vi "Main.vi"(11 "Module Admin":refnum<class "Delacor_lib_QMH_Module Admin.lvclass">) -> ()   [LabVIEW 2020, in "Sensor checking module.lvlib"]
doc: "This template is based off of the Queued Message Handler design pattern and the Queued Message Handler project template that ships with LabVIEW.\n\nThe main difference is that the queue is private to this module and communication between modules is performed via Broadcast and Request events.\n\nRequest events are wrapped in public API methods and are handled in the Event Handling Loop (EHL) of this VI. Any module can register for Broadcast events sent by this module. The EHL generates messages based on user interface actions.\n\nThe Message Handling Loop (MHL) processes messages generated by the EHL, or by other messages. The messages are string values, so new messages can be added easily to the Message Cases case structure in the MHL. Each message cluster can also provide an optional value for Message Data, which is a variant that can be converted to whatever message-specific data is required.\n_____\nBased on DQMH Project Template 7.0.1.1316."
uses:
  Sensor checking module.lvlib
  <vilib>/Delacor/Delacor QMH/Libraries/Module Admin_class/Delacor_lib_QMH_Module Admin.lvclass
  Module Data--cluster.ctl
  Simulated sensor signal HL Data.ctl
  <vilib>/Delacor/Delacor QMH/Libraries/Message Queue_class/Delacor_lib_QMH_Message Queue.lvclass/Delacor_lib_QMH_Message Queue.ctl
  Stop Argument--cluster.ctl
  <vilib>/Delacor/Delacor QMH/Libraries/Module Admin_class/Delacor_lib_QMH_Module Admin.lvclass/Delacor_lib_QMH_Module Admin.ctl
  Start sensor checking Argument--cluster.ctl
  Stop sensor checking Argument--cluster.ctl
  <vilib>/Utility/miscctls.llb/LVPointTypeDef.ctl
  <vilib>/Delacor/Delacor QMH/Libraries/Message Queue_class/Delacor_lib_QMH_Enqueue Message (Single).vi
  <vilib>/Delacor/Delacor QMH/Libraries/Module Admin_class/Delacor_lib_QMH_Get External Launch.vi
  <vilib>/Delacor/Delacor QMH/Libraries/Message Queue_class/Delacor_lib_QMH_Message Queue.lvclass
panel:
  out "error out":errorcluster
  out "Status":string
  in  "Simulate MHL Error":bool
  in  "Simulate EHL Error":bool
  # "Other processes communicate with this Module via its Public API (wrappers for its Request Events).\n\nThis Module communicates with other processes via its Broadcast Events.\nAny process that wants to receive these messages can register for this module's Broadcast events."
  # "This template is for the DQMH framework. See the block diagram for more information on how to use this template."
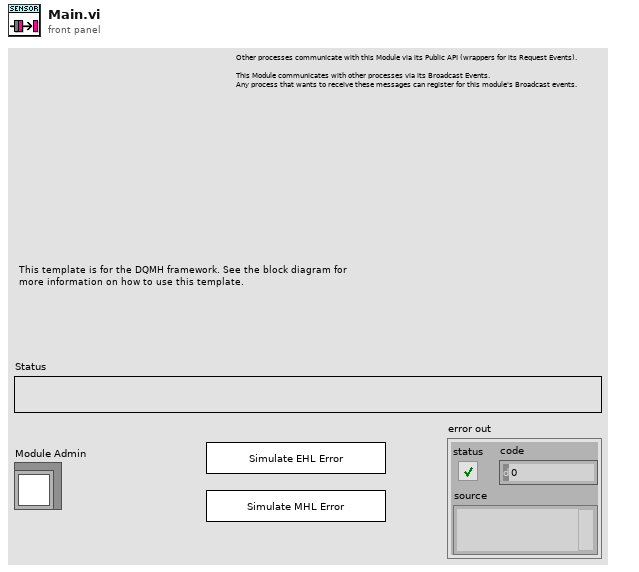
[diagram p1: front panel]
types:
  T1 = typedef "Sensor checking module.lvlib/Request Events--cluster.ctl" = cluster{"Stop Module":refnum<user-event>, "Show Panel":refnum<user-event>, "Hide Panel":refnum<user-event>, "Get Module Execution Status":refnum<user-event>, "Show Diagram":refnum<user-event>, "Start sensor checking":refnum<user-event>, "Stop sensor checking":refnum<user-event>, "Private":cluster{"Wake up HL":refnum<user-event>, "Sleep HL":refnum<user-event>}}
  T2 = typedef "Sensor checking module.lvlib/Simulated sensor signal HL Data.ctl" = cluster{"RPM increasing?":bool, "RPM":dbl}
  T3 = typedef "Sensor checking module.lvlib/Module Data--cluster.ctl" = cluster{"Status":string}
  T4 = enum32{"invalid lock state", "Not Locked", "Locked (No Password)", "Password-protected"}
  T5 = typedef "Sensor checking module.lvlib/Stop Argument--cluster.ctl" = cluster{"Origin":string, "Exit via Stop Module Req?":bool, "Wait for Module to stop?":bool}
  T6 = typedef "Sensor checking module.lvlib/Start sensor checking Argument--cluster.ctl" = cluster{"Triggered interval":dbl, "RPM increasing?":bool}
  T7 = typedef "Sensor checking module.lvlib/Stop sensor checking Argument--cluster.ctl" = cluster{"Boolean":bool}
  T8 = typedef "LVPointTypeDef.ctl" = cluster{"Horizontal":i16, "Vertical":i16}
  T9 = enum32{"Invalid", "Standard", "Closed", "Hidden", "Minimized", "Maximized"}
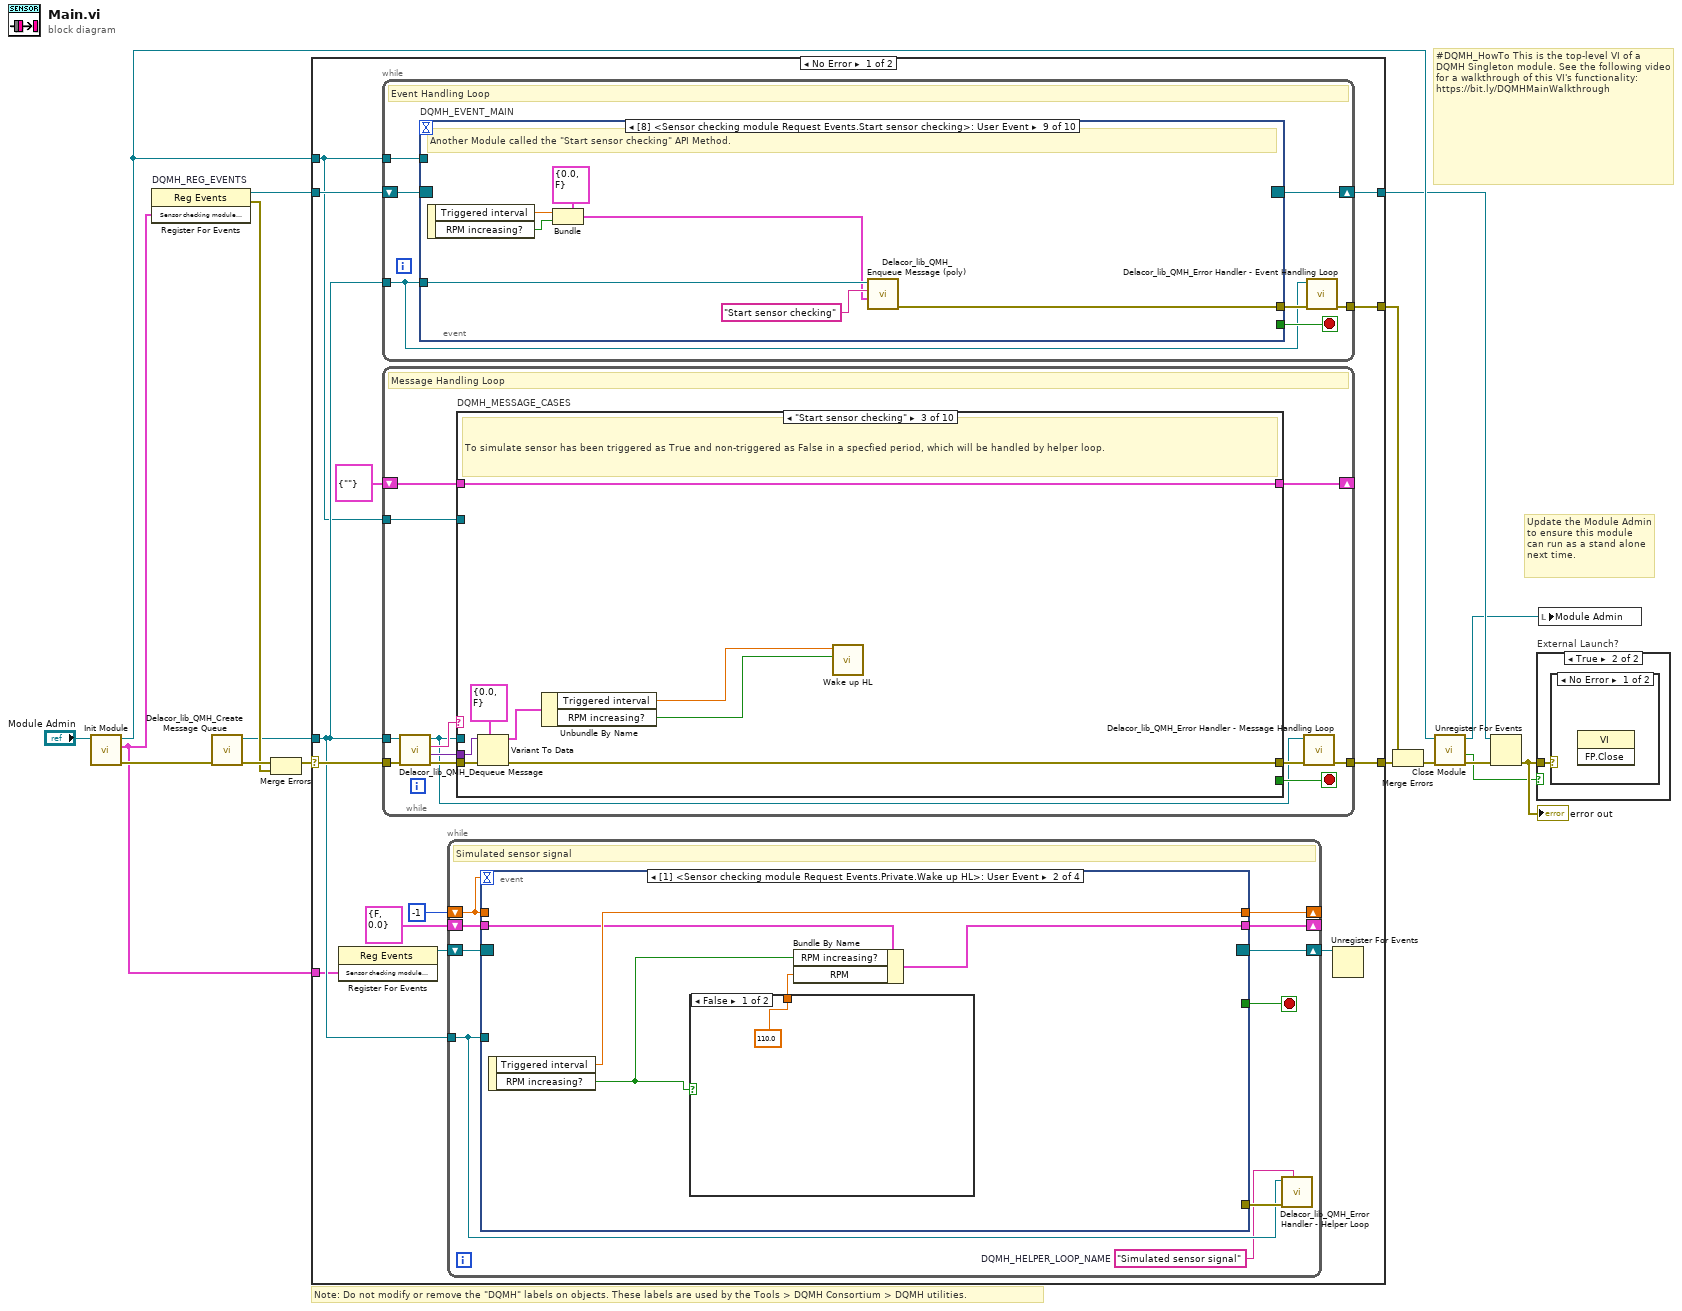
[diagram p0: block diagram]
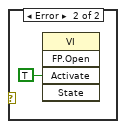
[diagram p3: hidden frame]
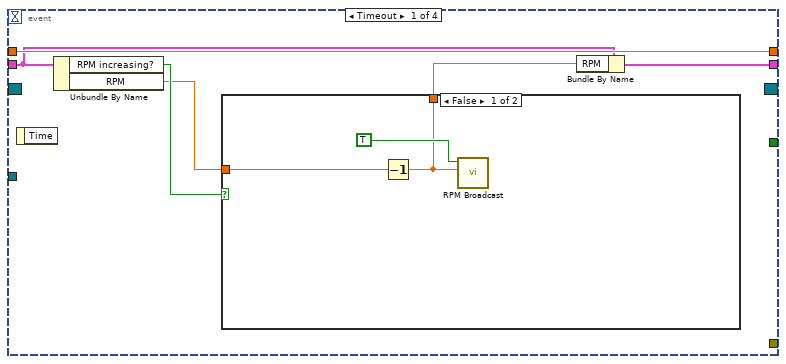
[diagram p4: hidden frame]
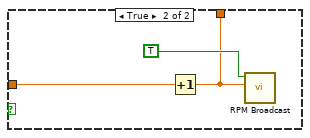
[diagram p5: hidden frame]
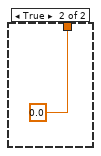
[diagram p6: hidden frame]
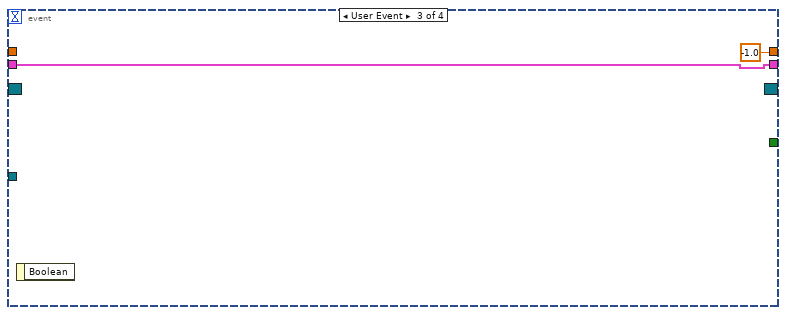
[diagram p7: hidden frame]
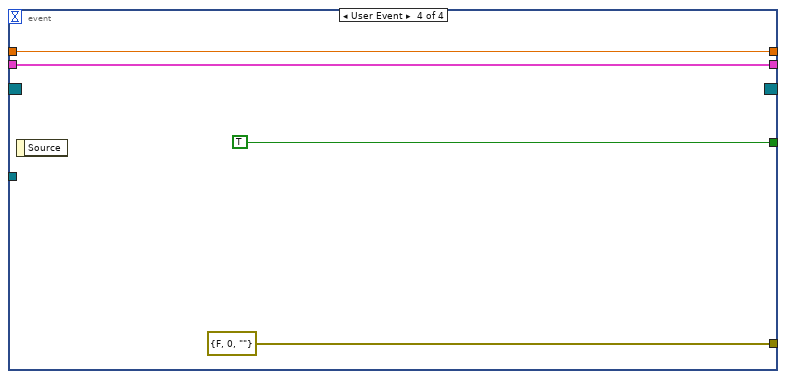
[diagram p8: hidden frame]
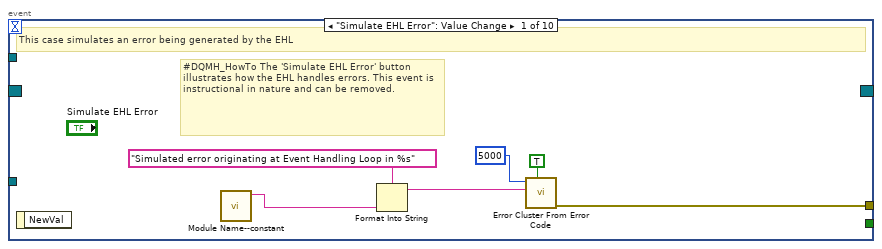
[diagram p9: hidden frame]
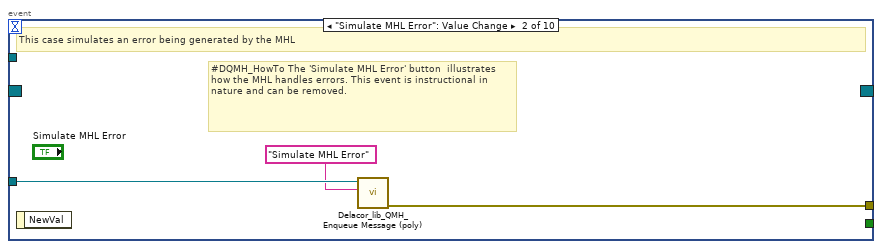
[diagram p10: hidden frame]
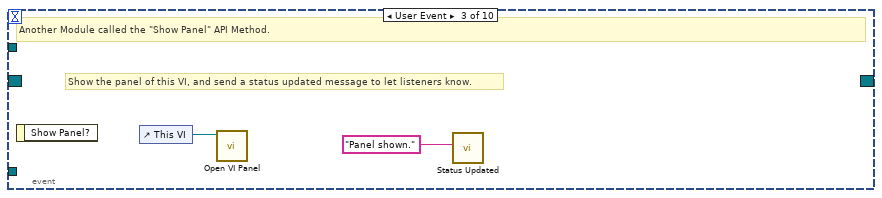
[diagram p11: hidden frame]
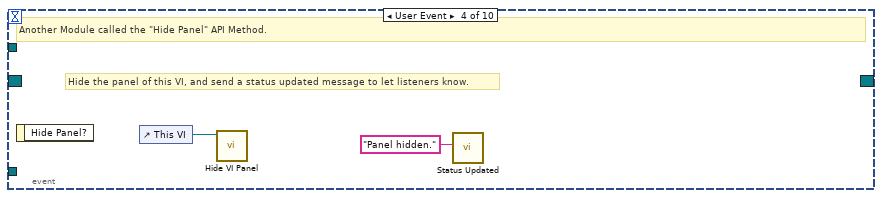
[diagram p12: hidden frame]
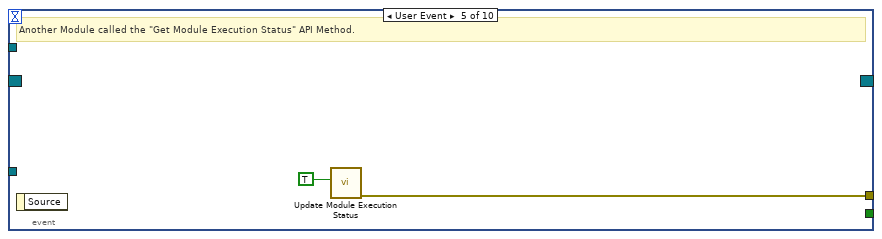
[diagram p13: hidden frame]
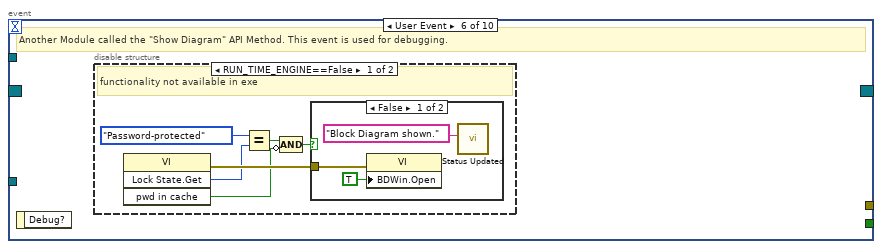
[diagram p14: hidden frame]
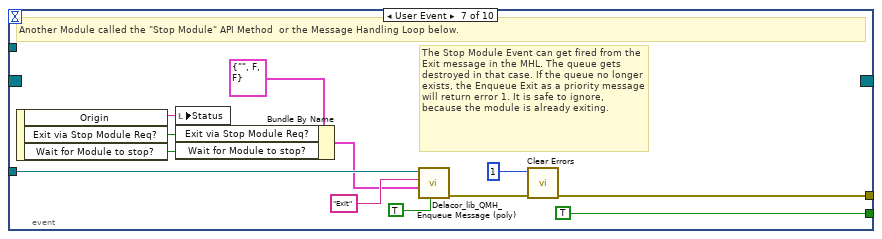
[diagram p17: hidden frame]
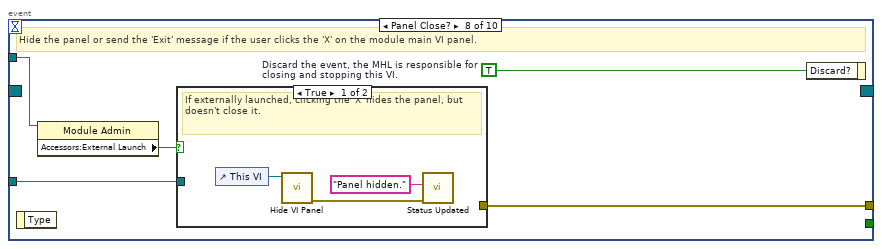
[diagram p18: hidden frame]
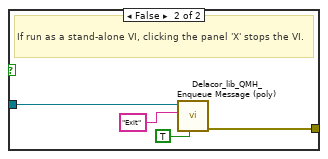
[diagram p19: hidden frame]
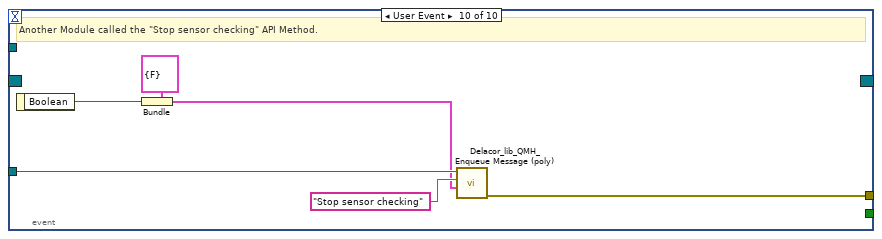
[diagram p20: hidden frame]
diagram:
  # "#DQMH_HowTo This is the top-level VI of a DQMH Singleton module. See the following video for a walkthrough of this VI's functionality: https://bit.ly/DQMHMainWalkthrough"
  # "Note: Do not modify or remove the \"DQMH\" labels on objects. These labels are used by the Tools > DQMH Consortium > DQMH utilities."
  # "Update the Module Admin to ensure this module can run as a stand alone next time."
  n1 = call "Init Module.vi"("Singleton Module Admin in"="Module Admin") -> ("error out"=w16:errorcluster, "Sensor checking module Request Events"=w1:T1, "Singleton Module Admin out"=w8:refnum<class "Delacor_lib_QMH_Module Admin.lvclass">)  [unwired: 8 in]
  n2 = register-events "DQMH_REG_EVENTS"(w1) -> (reference out=w6:refnum<event-registration>, error out=w9:errorcluster)  [unwired: 2 in]
  n3 = call <vilib>:"Delacor_lib_QMH_Create Message Queue.vi"("error in"=w16) -> ("error out"=w11:errorcluster, "Message Queue"=w5:refnum<class "Delacor_lib_QMH_Message Queue.lvclass">)  [unwired: 9 in]
  n4 = Merge Errors(w11, w9) -> (w10:errorcluster)
  n5 = case shown="No Error" w10 {
    selector: w10 -> [w28 w245]
    tunnel: [w30 w244] -> w17
    tunnel: [w27 w243] -> w7
    tunnel: w6 -> [w25 w243]
    tunnel: w5 -> [w24 w238]
    tunnel: [w29 _] -> w14
    tunnel: w8 -> [w23 w239]
    tunnel: w1 -> [w22 _]
    frame No Error {
      n6 = register-events ("DQMH_HELPER_REGFOREVENTS")(w22) -> (reference out=w20:refnum<event-registration>)  [unwired: 2 in, 1 out]
      n7 = while {
        tunnel: w24 -> [w66]
        shift-right: [w69] -> w27
        shift-left: w25 -> [w70]
        tunnel: [w71] -> w29
        tunnel: w23 -> [w67]
        stop <- w68 stop-if-true
        # "Event Handling Loop"
        n8 = event "DQMH_EVENT_MAIN" shown="[8] <Sensor checking module Request Events.Start sensor checking>: User Event" {
          selector: w70 -> [_ _ _ _ _ _ _ _ _ _]
          dyn-events: [_ _ _ _ _ _ _ _ _ _] -> w69
          timeout: _ -> [_ _ _ _ _ _ _ _ _ _]
          tunnel: [_ _ _ _ _ _ TRUE ("Discard?") _ _ _] -> w68
          tunnel: w66 -> [_ w80 _ _ _ _ w104 w111 w127 w133]
          tunnel: [w78 w81 _ _ w87 _ w107 w113 w122 w128] -> w72
          tunnel: w67 -> [_ _ _ _ _ _ _ w110 _ _]
          event "Simulate EHL Error": Value Change {
            # "#DQMH_HowTo The 'Simulate EHL Error' button  illustrates how the EHL handles errors. This event is instructional in nature and can be removed."
            # "This case simulates an error being generated by the EHL"
            n9 = event-data() -> ()  [unwired: 1 in, 1 out]
            n10 = call "Module Name--constant.vi"() -> ("Module Name"=w75:string)  [unwired: 11 in]
            n11 = Format Into String(format string="Simulated error originating at Event Handling Loop in %s", w75) -> (resulting string=w76:string)  [unwired: 2 in, 1 out]
            n12 = call <vilib>:"Error Cluster From Error Code.vi"("show call chain? (False)"=TRUE, "error message (\"\")"=w76, "error code (0)"=5000) -> ("error out"=w78:errorcluster)  [unwired: 6 in]
          }
          event "Simulate MHL Error": Value Change {
            # "#DQMH_HowTo The 'Simulate MHL Error' button  illustrates how the MHL handles errors. This event is instructional in nature and can be removed."
            # "This case simulates an error being generated by the MHL"
            n13 = event-data() -> ()  [unwired: 1 in, 1 out]
            n14 = call-poly <vilib>:"Delacor_lib_QMH_Enqueue Message (poly).vi"("Message"="Simulate MHL Error", "Message Queue in"=w80) -> ("error out"=w81:errorcluster)  [unwired: 8 in, 1 out]
          }
          event User Event {
            # "Show the panel of this VI, and send a status updated message to let listeners know."
            # "Another Module called the \"Show Panel\" API Method."
            n15 = event-data() -> ()  [unwired: 1 in, 1 out]
            n16 = control-ref of="This VI"() -> (w83:refnum<vi>)
            n17 = call "Open VI Panel.vi"("VI"=w83) -> ()  [unwired: 10 in, 1 out]
            n18 = call "Status Updated.vi"("Status"="Panel shown." ("format string")) -> ()  [unwired: 10 in, 1 out]
          }
          event User Event {
            # "Hide the panel of this VI, and send a status updated message to let listeners know."
            # "Another Module called the \"Hide Panel\" API Method."
            n19 = event-data() -> ()  [unwired: 1 in, 1 out]
            n20 = control-ref of="This VI"() -> (w85:refnum<vi>)
            n21 = call "Hide VI Panel.vi"("VI"=w85) -> ()  [unwired: 10 in, 1 out]
            n22 = call "Status Updated.vi"("Status"="Panel hidden." ("format string")) -> ()  [unwired: 10 in, 1 out]
          }
          event User Event {
            # "Another Module called the \"Get Module Execution Status\" API Method."
            n23 = event-data() -> ()  [unwired: 1 in, 1 out]
            n24 = call "Update Module Execution Status.vi"("Running?"=TRUE) -> ("error out"=w87:errorcluster)  [unwired: 10 in]
          }
          event User Event {
            # "Another Module called the \"Show Diagram\" API Method. This event is used for debugging."
            n25 = event-data() -> ()  [unwired: 1 in, 1 out]
            n26 = disable-structure shown="RUN_TIME_ENGINE==False" {
              frame condition #0 (active) {
                # "functionality not available in exe"
                n27 = invoke on="Invoke Node" class="VI" method="Lock State.Get"() -> (error out=w93:errorcluster, "Get Lock State"=w92:T4, "pwd in cache"=w89:bool)  [unwired: 4 in, 1 out]
                n28 = Equal?(x=T4."Password-protected", y=w92) -> (x = y?=w90:bool)
                n29 = Compound Arithmetic op=AND(w90, invert w89) -> (w88:bool)
                n30 = case shown="False" w88 {
                  tunnel: w93 -> [w96 _]
                  frame False {
                    n31 = property on="Property Node" class="VI"(error in=w96, "BDWin.Open"=TRUE ("Block Diagram Window:Open")) -> ()  [unwired: 1 in, 2 out]
                    n32 = call "Status Updated.vi"("Status"="Block Diagram shown." ("format string")) -> ()  [unwired: 10 in, 1 out]
                  }
                  frame True {
                    # "Password-protected VI, and the password is not in the cache. Do not show the diagram."
                  }
                }
              }
              frame condition #1 {
              }
            }
          }
          event User Event {
            # "The Stop Module Event can get fired from the Exit message in the MHL. The queue gets destroyed in that case. If the queue no longer exists, the Enqueue Exit as a priority message will return error 1. It is safe to ignore, because the module is already exiting."
            # "Another Module called the \"Stop Module\" API Method  or the Message Handling Loop below."
            n33 = event-data() -> ("Origin"=w103:string, "Exit via Stop Module Req?"=w99:bool, "Wait for Module to stop?"=w98:bool)  [unwired: 1 in]
            n34 = local write "Status"(w103) -> ()
            n35 = Bundle By Name(cluster=T5 {"Origin"="", "Exit via Stop Module Req?"=FALSE, "Wait for Module to stop?"=FALSE} ("Stop Argument"), "Exit via Stop Module Req?"=w99, "Wait for Module to stop?"=w98) -> (w97:T5)
            n36 = call-poly <vilib>:"Delacor_lib_QMH_Enqueue Message (poly).vi"("Priority Message? (F)"=TRUE, "Message Data"=w97, "Message"="Exit", "Message Queue in"=w104) -> ("error out"=w108:errorcluster)  [unwired: 6 in, 1 out]
            n37 = call <vilib>:"Clear Errors.vi"("error in (no error)"=w108, "specific error code to clear (0: all)"=1) -> ("error out"=w107:errorcluster)  [unwired: 4 in, 1 out]
          }
          event Panel Close? {
            w112 = TRUE  # Discard the event, the MHL is responsible for closing and stopping this VI.
            # "Hide the panel or send the 'Exit' message if the user clicks the 'X' on the module main VI panel."
            n38 = event-data() -> ()  [unwired: 1 in, 1 out]
            n39 = property on="Property Node" class="Module Admin"(reference=w110) -> ("Accessors:External Launch"=w109:bool)  [unwired: 1 in, 2 out]
            n40 = case shown="True" w109 {
              tunnel: w111 -> [_ w119]
              tunnel: [_ w120] -> w113
              frame True {
                # "If externally launched, clicking the 'X' hides the panel, but doesn't close it."
                n41 = control-ref of="This VI"() -> (w116:refnum<vi>)
                n42 = call "Hide VI Panel.vi"("VI"=w116) -> ("error out"=w114:errorcluster)  [unwired: 10 in]
                n43 = call "Status Updated.vi"("error in"=w114, "Status"="Panel hidden." ("format string")) -> ()  [unwired: 9 in, 1 out]
              }
              frame False {
                # "If run as a stand-alone VI, clicking the panel 'X' stops the VI."
                n44 = call-poly <vilib>:"Delacor_lib_QMH_Enqueue Message (poly).vi"("Priority Message? (F)"=TRUE, "Message"="Exit", "Message Queue in"=w119) -> ("error out"=w120:errorcluster)  [unwired: 7 in, 1 out]
              }
            }
            n45 = event-data ("Event Filter Node")("Discard?"=w112) -> ()  [unwired: 1 in, 1 out]
          }
          event User Event {
            # "Another Module called the \"Start sensor checking\" API Method."
            n46 = event-data() -> ("Triggered interval"=w123:dbl, "RPM increasing?"=w121:bool)  [unwired: 1 in]
            n47 = Bundle(cluster=T6 {"Triggered interval"=0.0, "RPM increasing?"=FALSE} ("Start sensor checking Argument"), "Triggered interval"=w123, "RPM increasing?"=w121) -> (w124:T6)
            n48 = call-poly <vilib>:"Delacor_lib_QMH_Enqueue Message (poly).vi"("Message Data"=w124, "Message"="Start sensor checking", "Message Queue in"=w127) -> ("error out"=w122:errorcluster)  [unwired: 7 in, 1 out]
          }
          event User Event {
            # "Another Module called the \"Stop sensor checking\" API Method."
            n49 = event-data() -> ("Boolean"=w129:bool)  [unwired: 1 in]
            n50 = Bundle(cluster=T7 {"Boolean"=FALSE} ("Stop sensor checking Argument"), "Boolean"=w129) -> (w130:T7)
            n51 = call-poly <vilib>:"Delacor_lib_QMH_Enqueue Message (poly).vi"("Message Data"=w130, "Message"="Stop sensor checking", "Message Queue in"=w133) -> ("error out"=w128:errorcluster)  [unwired: 7 in, 1 out]
          }
        }
        n52 = call-dynamic "Delacor_lib_QMH_Error Handler - Event Handling Loop.vi"("error in"=w72, "Message Queue in"=w66) -> ("dup error in"=w71:errorcluster)  [unwired: 8 in, 1 out]
      }
      n53 = while {
        tunnel: w24 -> [w134]
        shift-right: [w142] -> _
        shift-left: T3 {"Status"=""} ("Data Cluster") -> [w143]
        tunnel: w28 -> [w145]
        tunnel: [w137] -> w30
        tunnel: w23 -> [w138]
        stop <- w141 stop-if-true
        # "Message Handling Loop"
        n54 = call-dynamic "Delacor_lib_QMH_Dequeue Message.vi"("error in"=w145, "Message Queue in"=w134) -> ("error out"=w144:errorcluster, "Message Data"=w139:variant, "Message"=w140:string, "Message Queue out"=w135:refnum<class "Delacor_lib_QMH_Message Queue.lvclass">)  [unwired: 6 in]
        n55 = case "DQMH_MESSAGE_CASES" shown="\"Start sensor checking\"" w140 {
          selector: w140 -> [_ _ _ _ _ _ _ _ _ w233]
          tunnel: w135 -> [_ _ _ _ _ _ _ w199 w221 _]
          tunnel: w144 -> [w163 w167 w175 w181 w184 w186 w195 w206 w227 w236]
          tunnel: [w161 w167 w173 w179 w183 w186 w194 w202 w222 w237] -> w136
          tunnel: w143 -> [w152 w166 w174 w180 w182 w185 w192 w201 w220 w234]
          tunnel: [w151 w166 w174 w180 w182 w185 w192 w201 w220 w234] -> w142
          tunnel: [_ _ _ _ _ _ _ _ w219 _] -> w141
          tunnel: w139 -> [_ _ w172 w178 _ _ _ w200 w218 _]
          tunnel: w138 -> [w153 _ _ _ _ _ _ w198 w213 _]
          frame "Initialize" {
            w147 = "Initial Message" ("Initial Message")
            # "#CodeNeeded - Initialize the appearance of the front panel."
            # "#CodeNeeded - Initialize your state data here."
            # "Initialize - Any operation that needs to be done before the module can receive messages. Synchronize Caller Events.vi will inform Start Module.vi that the module has launched and is ready to receive messages. Module Did Init.vi will broadcast that the module initialized."
            n56 = call "Synchronize Caller Events.vi"("error in"=w163, "Singleton Module Admin in"=w153) -> ("error out"=w162:errorcluster, "Singleton Module Admin out"=w148:refnum<class "Delacor_lib_QMH_Module Admin.lvclass">)  [unwired: 8 in]
            n57 = property on="Property Node" class="Module Admin"(reference=w148) -> ("Accessors:External Launch"=w157:bool)  [unwired: 1 in, 2 out]
            n58 = Select(t=T9."Hidden" ("State"), s=w157, f=T9."Standard" ("State")) -> (s? t:f=w154:T9)
            n59 = call "Module Name--constant.vi"() -> ("Module Name"=w160:string)  [unwired: 11 in]
            n60 = property on="Property Node" class="VI"("Front Panel.Title"=w160) -> (reference out=w159:refnum<vi>, error out=w165:errorcluster)  [unwired: 2 in]
            n61 = call "Module Name--constant.vi"() -> ("Module Name"=w149:string)  [unwired: 11 in]
            n62 = invoke on="Invoke Node" class="VI" method="FP.Open"(reference=w159, error in=w165, "State"=w154) -> (reference out=w158:refnum<vi>, error out=w164:errorcluster)  [unwired: 2 in, 3 out]
            n63 = Bundle By Name(cluster=w152, "Status"=w147) -> (w151:T3)
            n64 = call "Module Did Init.vi"("error in"=w162, "Initialized?"=TRUE, "Origin"=w149) -> ("error out"=w161:errorcluster)  [unwired: 8 in]
            n65 = invoke on="Invoke Node" class="VI" method="FP.Center"(reference=w158, error in=w164) -> ()  [unwired: 1 in, 3 out]
            n66 = property on="Pane" class="Pane"("Origin"=T8 {"Horizontal"=0, "Vertical"=0}) -> ()  [unwired: 2 in, 2 out]
            "Status" <- w147
          }
          frame "---Module Specific---" {
            # "Separator -- The following cases handle messages specific to this Module."
          }
          frame "Start sensor checking" {
            # "To simulate sensor has been triggered as True and non-triggered as False in a specfied period, which will be handled by helper loop."
            n67 = Variant To Data(error in=w175, type=T6 {"Triggered interval"=0.0, "RPM increasing?"=FALSE} ("Start sensor checking Argument"), Variant=w172) -> (data=w170:T6, error out=w173:errorcluster)
            n68 = Unbundle By Name(w170) -> ("Triggered interval"=w169:dbl, "RPM increasing?"=w168:bool)
            n69 = call "Wake up HL.vi"("Triggered interval"=w169, "RPM increasing?"=w168) -> ()  [unwired: 7 in, 1 out]
          }
          frame "Stop sensor checking" {
            # "To stop simulating sensor has been triggering and non-triggered, which will let helper loop to sleep."
            n70 = Variant To Data(error in=w181, type=T7 {"Boolean"=FALSE} ("Stop sensor checking Argument"), Variant=w178) -> (data=w176:T7, error out=w179:errorcluster)
            n71 = Unbundle By Name(w176) -> ()  [unwired: 1 out]
            n72 = call "Sleep HL.vi"() -> ()  [unwired: 11 in, 1 out]
          }
          frame "---Copy This Frame---" {
            # "Duplicate this frame when creating new messages.  Change this comment in the duplicated frame to describe this message."
            n73 = Merge Errors(w184) -> (w183:errorcluster)
          }
          frame "---Exit and Error Handling---" {
            # "Separator - The following cases handle errors and exit messages."
          }
          frame "Simulate MHL Error" {
            # "#DQMH_HowTo The 'Simulate MHL Error' button  illustrates how the MHL handles errors. This event is instructional in nature and can be removed."
            # "Simulate an error occurring at the MHL"
            n74 = call "Module Name--constant.vi"() -> ("Module Name"=w188:string)  [unwired: 11 in]
            n75 = Format Into String(format string="Simulated error originating at Message Handling Loop in %s", w188) -> (resulting string=w189:string)  [unwired: 2 in, 1 out]
            n76 = call <vilib>:"Error Cluster From Error Code.vi"("show call chain? (False)"=TRUE, "error message (\"\")"=w189, "error code (0)"=5001) -> ("error out"=w193:errorcluster)  [unwired: 6 in]
            n77 = Merge Errors(w195, w193) -> (w194:errorcluster)
          }
          frame "Error" {
            # "#CodeRecommended - If the module is running in standalone mode (External Launch = FALSE), this code will pop up an error dialog and call the 'Exit' message if an error occurs. Add more fine-grained error management here."
            # "Error - Check the error message data and respond accordingly. This message is sent by the \"Error Handler\" VIs at the end of each loop in this application."
            n78 = property on="Property Node" class="Module Admin"(reference=w198) -> ("Accessors:External Launch"=w197:bool)  [unwired: 1 in, 2 out]
            n79 = Variant To Data(error in=w206, type=errorcluster {"status"=FALSE, "code"=0, "source"=""} ("error constant"), Variant=w200) -> (data=w196:errorcluster, error out=w204:errorcluster)
            n80 = local write "error out"(w196) -> ()
            n81 = call "Error Reported.vi"("Error"=w196) -> ()  [unwired: 10 in, 1 out]
            n82 = case shown="False" w197 {
              tunnel: [w211 _] -> w203
              tunnel: w199 -> [w209 _]
              tunnel: w196 -> [w210 _]
              frame False {
                n83 = disable-structure shown="Default" {
                  disable-tunnel: w210 -> [w212 _]
                  frame condition #0 (active) {
                    # "If the module is running standalone, then pop up an error dialog and call the \"Exit\" message."
                    n84 = call <vilib>:"Simple Error Handler.vi"("error in (no error)"=w212) -> ()  [unwired: 4 in, 5 out]
                  }
                  frame condition #1 {
                    # "To prevent the Simple Error Handler VI from being loaded (e.g. when deploying to a Real-Time target), add the Conditional Disable Symbol \"DQMH_Disable_SEH\" to your project and set it to TRUE."
                  }
                }
                n85 = call-poly <vilib>:"Delacor_lib_QMH_Enqueue Message (poly).vi"("Priority Message? (F)"=TRUE, "Message"="Exit", "Message Queue in"=w209) -> ("error out"=w211:errorcluster)  [unwired: 7 in, 1 out]
              }
              frame True {
                # "If the module was launched externally, calling the Error Reported broadcast VI is the only action performed by the \"Error\" message. The module's caller can then process the error appropriately."
              }
            }
            n86 = Merge Errors(w204, w203) -> (w202:errorcluster)
          }
          frame "Exit" {
            w217 = 91  # 91: not all Exit messages will have an argument
            w219 = TRUE  # Stop the VI
            # "Release the message queue reference"
            # "#CodeNeeded - Add any required cleanup code here."
            # "Exit - Exit the application."
            n87 = Variant To Data(error in=w227, type=T5 {"Origin"="", "Exit via Stop Module Req?"=FALSE, "Wait for Module to stop?"=FALSE} ("Stop Argument"), Variant=w218) -> (data=w215:T5, error out=w224:errorcluster)
            n88 = call <vilib>:"Clear Errors.vi"("error in (no error)"=w224, "specific error code to clear (0: all)"=w217) -> ("error out"=w226:errorcluster)  [unwired: 4 in, 1 out]
            n89 = control-ref of="This VI"() -> (w214:refnum<vi>)
            n90 = call-dynamic "Delacor_lib_QMH_Release Message Queue.vi"("error in"=w226, "Message Queue"=w221) -> ("error out"=w225:errorcluster)  [unwired: 9 in]
            n91 = call "Handle Exit.vi"("Stop Argument"=w215, "Admin in"=w213, "VI reference"=w214) -> ("error out"=w223:errorcluster)  [unwired: 7 in, 1 out]
            n92 = Merge Errors(w225, w223) -> (w222:errorcluster)
            n93 = call "Error Reported.vi"("Error"=w222) -> ()  [unwired: 10 in, 1 out]
          }
          frame Default {
            # "'Default' case only runs if there is a message that isn't defined in any of the other cases.  Output a programming error."
            n94 = call "Module Name--constant.vi"() -> ("Module Name"=w232:string)  [unwired: 11 in]
            n95 = Format Into String(format string="The invalid message string \"%s\" was received in the Message Handling Loop for module \"%s\".", w233, w232) -> (resulting string=w228:string)  [unwired: 2 in, 1 out]
            n96 = call <vilib>:"Error Cluster From Error Code.vi"("show call chain? (False)"=TRUE, "error message (\"\")"=w228, "error code (0)"=1) -> ("error out"=w235:errorcluster)  [unwired: 6 in]
            n97 = Merge Errors(w236, w235) -> (w237:errorcluster)
          }
        }
        n98 = call-dynamic "Delacor_lib_QMH_Error Handler - Message Handling Loop.vi"("error in"=w136, "Message Queue in"=w135) -> ("dup error in"=w137:errorcluster)  [unwired: 8 in, 1 out]
      }
      n99 = while "DQMH_HELPER_LOOP" {
        shift-right: [w40] -> _
        shift-left: -1 -> [w39]
        shift-right: [w37] -> w21
        shift-left: w20 -> [w38]
        tunnel: w24 -> [w34]
        shift-right: [w31] -> _
        shift-left: T2 {"RPM increasing?"=FALSE, "RPM"=0.0} ("Simulated sensor signal HL Data") -> [w32]
        stop <- w36 stop-if-true
        w33 = "Simulated sensor signal"  # DQMH_HELPER_LOOP_NAME
        # "Simulated sensor signal"
        n100 = event "DQMH_HELPER_EVENT_STRUCTURE" shown="[1] <Sensor checking module Request Events.Private.Wake up HL>: User Event" {
          selector: w38 -> [_ _ _ _]
          dyn-events: [_ _ _ _] -> w37
          timeout: w39 -> [_ _ _ _]
          tunnel: w39 -> [w46 _ _ w65]
          tunnel: [w46 w57 -1.0 ("Triggered interval") w65] -> w40
          tunnel: [_ _ _ TRUE] -> w36
          tunnel: [_ _ _ errorcluster {"status"=FALSE, "code"=0, "source"=""} ("error constant")] -> w35
          tunnel: w34 -> [_ _ _ _]
          tunnel: [w42 w56 w60 w62] -> w31
          tunnel: w32 -> [w43 w55 w60 w62]
          event Timeout {
            n101 = event-data() -> ()  [unwired: 1 in, 1 out]
            n102 = Unbundle By Name(w43) -> ("RPM increasing?"=w45:bool, "RPM"=w44:dbl)
            n103 = case shown="False" w45 {
              tunnel: w44 -> [w47 w51]
              tunnel: [w48 w50] -> w41
              frame False {
                n104 = Decrement(x=w47) -> (x-1=w48:dbl)
                n105 = call "RPM Broadcast.vi"("Triggered?"=TRUE, "RPM"=w48) -> ()  [unwired: 8 in, 1 out]
              }
              frame True {
                n106 = Increment(x=w51) -> (x+1=w50:dbl)
                n107 = call "RPM Broadcast.vi"("Triggered?"=TRUE, "RPM"=w50) -> ()  [unwired: 8 in, 1 out]
              }
            }
            n108 = Bundle By Name(cluster=w43, "RPM"=w41) -> (w42:T2)
          }
          event User Event {
            n109 = event-data() -> ("Triggered interval"=w57:dbl, "RPM increasing?"=w54:bool)  [unwired: 1 in]
            n110 = case shown="False" w54 {
              tunnel: [110.0 ("Start RPM") 0.0 ("Start RPM")] -> w53
              frame False {
              }
              frame True {
              }
            }
            n111 = Bundle By Name(cluster=w55, "RPM increasing?"=w54, "RPM"=w53) -> (w56:T2)
          }
          event User Event {
            n112 = event-data() -> ()  [unwired: 1 in, 1 out]
          }
          event User Event {
            n113 = event-data() -> ()  [unwired: 1 in, 1 out]
          }
        }
        n114 = call-dynamic "Delacor_lib_QMH_Error Handler - Helper Loop.vi"("Error Debug"=w33, "error in"=w35, "Message Queue in"=w34) -> ()  [unwired: 7 in, 2 out]
      }
      n115 = Unregister For Events(event registration refnum=w21) -> ()  [unwired: 1 in, 1 out]
    }
    frame Error {
      # "Synchronize Caller Events.vi will inform Start Module.vi that the module has launched and will let the code calling Start Module.vi register for broadcasts and would permit the caller receive the broadcast that an error occurred at launch time."
      n116 = call-dynamic "Delacor_lib_QMH_Release Message Queue.vi"("error in"=w245, "Message Queue"=w238) -> ("error out"=w244:errorcluster)  [unwired: 9 in]
      n117 = call "Synchronize Caller Events.vi"("Singleton Module Admin in"=w239) -> ("error out"=w246:errorcluster)  [unwired: 9 in, 1 out]
      n118 = call "Module Name--constant.vi"() -> ("Module Name"=w242:string)  [unwired: 11 in]
      n119 = Format Into String(format string="An error occurred during initialization. %s is no longer running.", w242) -> (resulting string=w240:string)  [unwired: 2 in, 1 out]
      n120 = Merge Errors(w244, w246) -> (w247:errorcluster)
      n121 = call "Error Reported.vi"("Additional Information"=w240, "Error"=w247) -> ()  [unwired: 9 in, 1 out]
    }
  }
  n122 = Merge Errors(w14, w17) -> (w13:errorcluster)
  n123 = call "Close Module.vi"("error in"=w13, "Module Admin in"=w8) -> ("error out"=w15:errorcluster, "External Launch"=w2:bool, "Module Admin out"=w3:refnum<class "Delacor_lib_QMH_Module Admin.lvclass">)  [unwired: 7 in]
  n124 = Unregister For Events(event registration refnum=w7, error in=w15) -> (error out=w12:errorcluster)
  "error out" <- w12
  n125 = case "External Launch?" shown="True" w2 {
    tunnel: w12 -> [_ w248]
    frame False {
    }
    frame True {
      n126 = case shown="No Error" w248 {
        frame No Error {
          n127 = invoke on="Invoke Node" class="VI" method="FP.Close"() -> ()  [unwired: 3 in, 3 out]
        }
        frame Error {
          n128 = invoke on="Invoke Node" class="VI" method="FP.Open"("Activate"=TRUE ("Activate?")) -> ()  [unwired: 4 in, 5 out]
        }
      }
    }
  }
  n129 = local write "Module Admin"(w3) -> ()
